vi "Write Teller In Msg.vi"(6 "Teller Metadata":refnum<class "Teller Metadata.lvclass">, 7 "Msg in":refnum<class "Msg.lvclass">, 9 "Relation":T1, 10 "Attributes":refnum<class "Attributes.lvclass">) -> (5 "Msg out":refnum<class "Msg.lvclass">)   [LabVIEW 2025, in "jettl.lvlib"]
uses:
  jettl.lvlib
  Msg/Msg.lvclass
  Relation.ctl
  Attributes/Attributes.lvclass
  Teller Metadata/Teller Metadata.lvclass
  Msg Input/Msg Input.lvclass
  Base Teller/Base Teller.lvlib
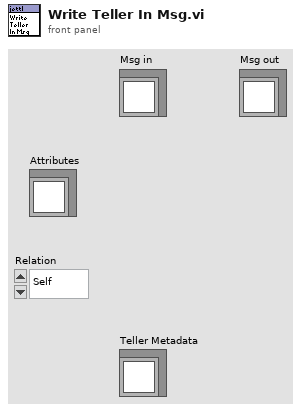
[diagram p1: front panel]
types:
  T1 = typedef "jettl.lvlib/Relation.ctl" = enum16{"Self", "Parent", "Child", "No Relation"}
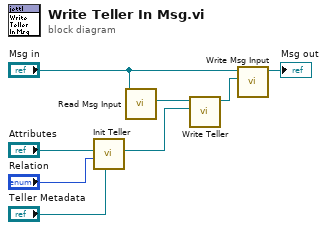
[diagram p0: block diagram]
diagram:
  n1 = call "Init Teller.vi"("Teller Metadata"="Teller Metadata", "Relation"="Relation", "Attributes"="Attributes") -> ("Teller"=w6:refnum<class "Teller.lvclass">)  [unwired: 8 in]
  n2 = call-dynamic "Read Msg Input.vi"("Msg in"="Msg in") -> ("Msg Input"=w8:refnum<class "Msg Input.lvclass">)  [unwired: 10 in]
  n3 = call-dynamic "Write Teller.vi"("Teller"=w6, "Msg Input in"=w8) -> ("Msg Input out"=w7:refnum<class "Msg Input.lvclass">)  [unwired: 9 in]
  n4 = call-dynamic "Write Msg Input.vi"("Msg Input"=w7, "Msg in"="Msg in") -> ("Msg out"=→"Msg out":refnum<class "Msg.lvclass">)  [unwired: 9 in]
